vi "FPGA_fast cycles-4.vi"() -> ()   [LabVIEW 2010]
uses:
  fast cycles/FPGA_run-states.ctl
  <vilib>/rvi/DataTransferAndStorage/Container/XNode/niFpgaContainer.xnode
  <vilib>/eio/EIONode/EIONode.xnode
  <vilib>/rvi/eio/nirviEIOImplementation/nirviEIOImplementation.xnode
  <vilib>/rvi/eio/common/nirviEmuClasses.ctl
  <vilib>/rvi/FIFO/Fifo_Resource/nirvififoEmulationSetSize.vi
  <vilib>/rvi/DataTransferAndStorage/Container/Common/niFpgaContainerGetUniqueNameForEmu.vi
  <vilib>/rvi/Memory/Memory_Emulation/nirvimemoryEmulationManagerCache_GetValue.vi
  <vilib>/rvi/Memory/Memory_Emulation/nirvimemoryEmulationManagerCache_InsertValue.vi
  <vilib>/Utility/error.llb/Clear Errors.vi
  <vilib>/rvi/Memory/Memory_Emulation/nirvimemoryEmulationManagerCache_SetValue.vi
  <vilib>/rvi/eio/common/nirviEmuTemplateMethod_noerrors.vi
panel:
  out "ramp":bool
  out "trigDAC":bool
  in  "order in":u64=360850920143060992
  in  "get order":bool
  in  "Stop seq 2":bool=TRUE
  in  "stop on sample count":bool
  in  "samples":u16=1
  in  "pulse length":u16=100
  in  "Divider":u32=200000
  out "voltmeters trig":bool=TRUE
  in  "Stop seq":bool=TRUE
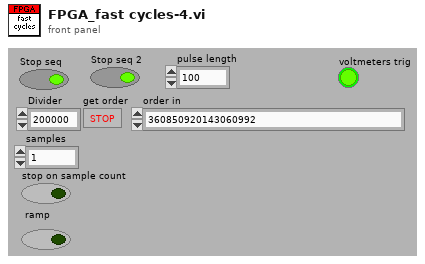
[diagram p1: front panel]
types:
  T1 = typedef "FPGA_run-states.ctl" = enum16{"stopped", "check", "reserve", "run", "release"}
  T2 = typedef "nirviEmuClasses.ctl" = enum16{"IO Read", "IO Write", "Method", "Property Read", "Property Write"}
  T3 = cluster{"Boolean array[0]":bool, "Boolean array[1]":bool, "Boolean array[2]":bool, "Boolean array[3]":bool, "Boolean array[4]":bool, "Boolean array[5]":bool, "Boolean array[6]":bool, "Boolean array[7]":bool, "Boolean array[8]":bool, "Boolean array[9]":bool, "Boolean array[10]":bool, "Boolean array[11]":bool, "Boolean array[12]":bool, "Boolean array[13]":bool, "Boolean array[14]":bool, "Boolean array[15]":bool}
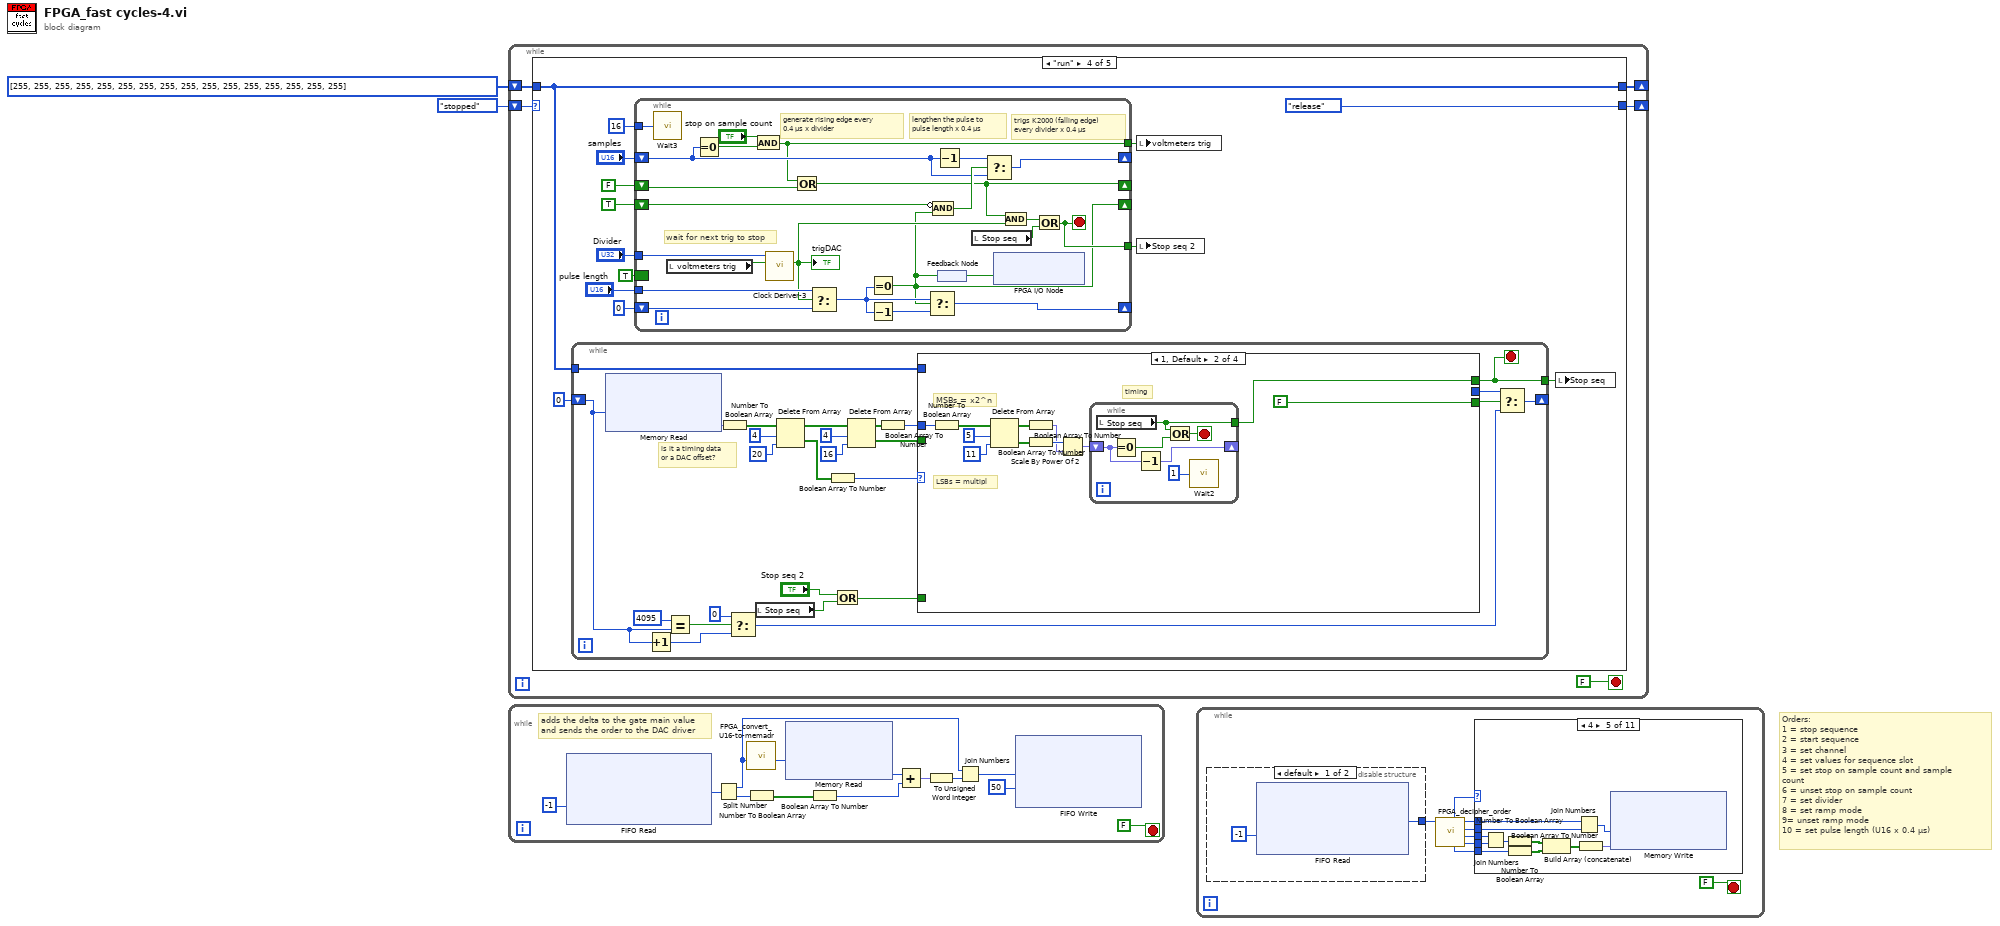
[diagram p0: block diagram]
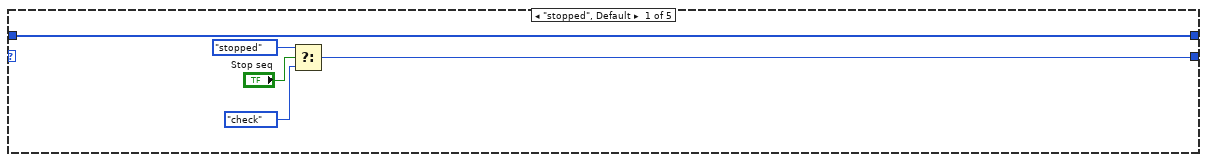
[diagram p2: hidden frame]
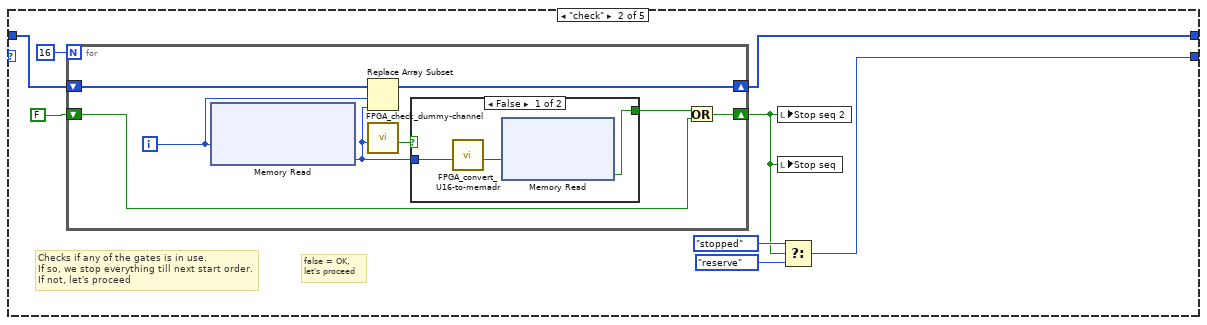
[diagram p3: hidden frame]
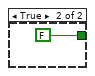
[diagram p4: hidden frame]
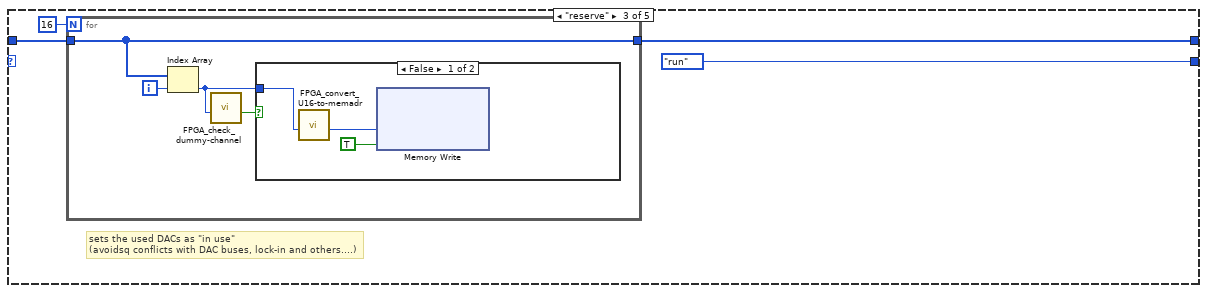
[diagram p5: hidden frame]
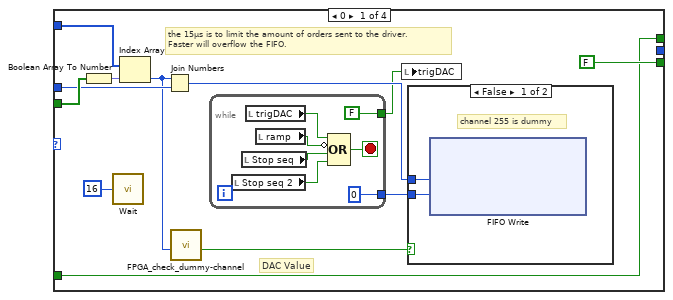
[diagram p7: hidden frame]
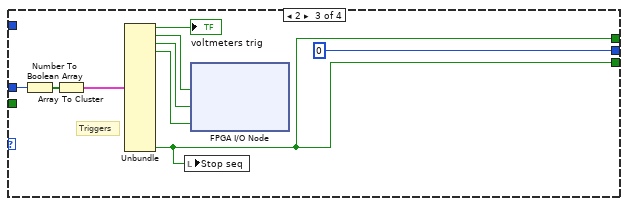
[diagram p9: hidden frame]
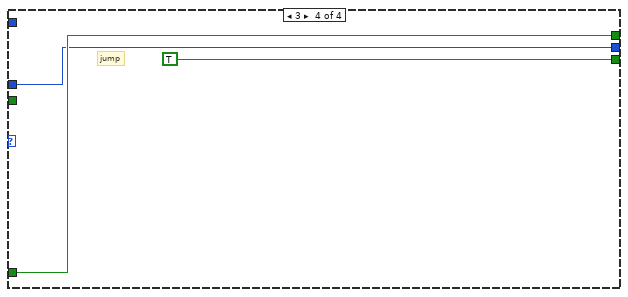
[diagram p10: hidden frame]
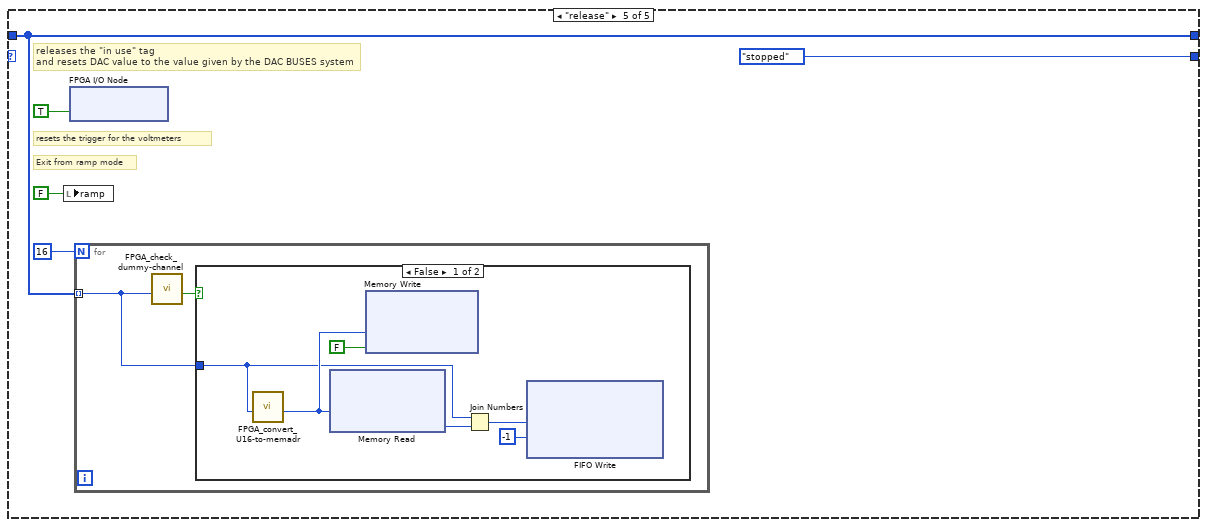
[diagram p11: hidden frame]
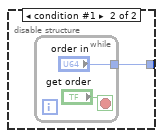
[diagram p13: hidden frame]
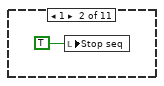
[diagram p15: hidden frame]
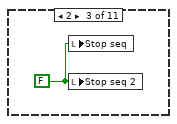
[diagram p16: hidden frame]
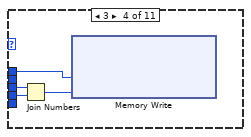
[diagram p17: hidden frame]
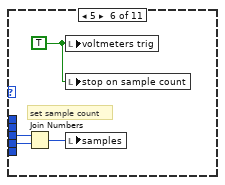
[diagram p18: hidden frame]
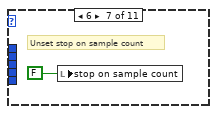
[diagram p19: hidden frame]
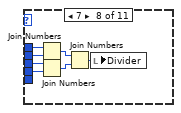
[diagram p20: hidden frame]
diagram:
  # "Orders:\n1 = stop sequence\n2 = start sequence\n3 = set channel\n4 = set values for sequence slot\n5 = set stop on sample count and sample count\n6 = unset stop on sample count\n7 = set divider\n8 = set ramp mode\n9= unset ramp mode\n10 = set pulse length (U16 x 0.4 µs)"
  n1 = while {
    shift-right: [w5] -> _
    shift-left: FPGA_run-states."stopped" ("run states") -> [w6]
    shift-right: [w3] -> _
    shift-left: u16[] [255, 255, 255, 255, 255, 255, 255, 255, 255, 255, 255, 255, 255, 255, 255, 255] -> [w4]
    stop <- FALSE stop-if-true
    n2 = case shown="\"run\"" w6 {
      tunnel: [w9 w13 FPGA_run-states."run" ("run states") FPGA_run-states."release" ("run states") FPGA_run-states."stopped" ("run states")] -> w5
      tunnel: [w8 w14 w285 w424 w757] -> w3
      tunnel: w4 -> [w8 w15 w286 w424 w757]
      frame "stopped", Default {
        n3 = Select(t=FPGA_run-states."stopped" ("run states"), s="Stop seq", f=FPGA_run-states."check" ("run states")) -> (s? t:f=w9:T1)
      }
      frame "check" {
        # "Checks if any of the gates is in use.\nIf so, we stop everything till next start order.\nIf not, let's proceed"
        # "false = OK,\nlet's proceed"
        n4 = for {
          N: 16 -> [_]
          shift-right: [w26] -> w16
          shift-left: FALSE ("Data") -> [w25]
          shift-right: [w24] -> w14
          shift-left: w15 -> [w23]
          i -> [w28]
          n5 = xnode ("Memory Read")("Address"=w28) -> ("Data"=w21:u16)  [unwired: 1 in, 1 out]
          n6 = Replace Array Subset(array=w23, new element=w21, index=w28) -> (w24:u16[])
          n7 = call "FPGA_check_dummy-channel.vi"("pan-channel"=w21) -> ("dummy?"=w22:bool)  [unwired: 10 out]
          n8 = case shown="False" w22 {
            tunnel: w21 -> [w157 _]
            tunnel: [w155 FALSE ("Data")] -> w27
            frame False {
              n9 = call "FPGA_convert_U16-to-memadr.vi"("Numeric"=w157) -> ("mem adr"=w156:u8)  [unwired: 10 out]
              n10 = xnode ("Memory Read")("Address"=w156) -> ("Data"=w155:bool)  [unwired: 1 in, 1 out]
            }
            frame True {
            }
          }
          n11 = Or(x=w27, y=w25) -> (x .or. y?=w26:bool)
        }
        n12 = local write "Stop seq 2"(w16) -> ()
        n13 = local write "Stop seq"(w16) -> ()
        n14 = Select(t=FPGA_run-states."stopped" ("run states"), s=w16, f=FPGA_run-states."reserve" ("run states")) -> (s? t:f=w13:T1)
      }
      frame "reserve" {
        # "sets the used DACs as \"in use\"\n(avoidsq conflicts with DAC buses, lock-in and others....)"
        n15 = for {
          N: 16 -> [_]
          tunnel: w286 -> [w291]
          tunnel: [w291] -> w285
          i -> [w292]
          n16 = Index Array(array=w291, index=w292) -> (element=w290:u16)
          n17 = call "FPGA_check_dummy-channel.vi"("pan-channel"=w290) -> ("dummy?"=w289:bool)  [unwired: 10 out]
          n18 = case shown="False" w289 {
            tunnel: w290 -> [w293 _]
            frame False {
              n19 = call "FPGA_convert_U16-to-memadr.vi"("Numeric"=w293) -> ("mem adr"=w295:u8)  [unwired: 10 out]
              n20 = xnode ("Memory Write")("Address"=w295, "Data"=TRUE) -> ()  [unwired: 1 in, 1 out]
            }
            frame True {
            }
          }
        }
      }
      frame "run" {
        n21 = while {
          shift-right: [w478] -> _
          shift-left: u16 0 ("t") -> [w490]
          tunnel: [w471] -> w426
          tunnel: w424 -> [w470]
          stop <- w471 stop-if-true
          # "is it a timing data\nor a DAC offset?"
          n22 = xnode ("Memory Read")("Address"=w490) -> ("Data"=w489:fxp<+,24,24>)  [unwired: 1 in, 1 out]
          n23 = Increment(x=w490) -> (x+1=w492:u16)
          n24 = Equal?(x=u16 4095, y=w490) -> (x = y?=w494:bool)
          n25 = Number To Boolean Array(number=w489) -> (Boolean array=w488:bool[])
          n26 = Select(t=u16 0, s=w494, f=w492) -> (s? t:f=w491:u16)
          n27 = local read "Stop seq"() -> (w475:bool)
          n28 = Delete From Array(array=w488, length=4, index=20) -> (deleted portion=w481:bool[], array with subset deleted=w485:bool[])
          n29 = Boolean Array To Number(Boolean array=w481) -> (number=w479:u8)
          n30 = Or(x="Stop seq 2", y=w475) -> (x .or. y?=w473:bool)
          n31 = Delete From Array(array=w485, length=4, index=16) -> (deleted portion=w482:bool[], array with subset deleted=w483:bool[])
          n32 = Boolean Array To Number(Boolean array=w483) -> (number=w474:u16)
          n33 = case shown="1, Default" w479 {
            tunnel: w474 -> [w631 w704 w719 w753]
            tunnel: w482 -> [w633 _ _ _]
            tunnel: [FALSE ("Stop seq") FALSE ("Stop seq") w713 TRUE ("Stop seq")] -> w477
            tunnel: [_ _ u16 0 w753] -> w476
            tunnel: [w627 w694 w713 w754] -> w471
            tunnel: w473 -> [w627 _ _ w754]
            tunnel: w470 -> [w625 _ _ _]
            frame 0 {
              # "the 15µs is to limit the amount of orders sent to the driver.\nFaster will overflow the FIFO."
              # "DAC Value"
              n34 = Boolean Array To Number(Boolean array=w633) -> (number=w632:fxp<+,4,4>)
              n35 = call "Wait"("Count(uSec)"=u8 16) -> ()  [unwired: 1 out]
              n36 = Index Array(array=w625, index=w632) -> (element=w623:u16)
              n37 = Join Numbers(hi=w623, lo=w631) -> ((hi.lo)=w630:u32)
              n38 = call "FPGA_check_dummy-channel.vi"("pan-channel"=w623) -> ("dummy?"=w624:bool)  [unwired: 10 out]
              n39 = while {
                tunnel: [0 ("Timeout")] -> w626
                tunnel: [FALSE ("Stop seq 3")] -> w622
                stop <- w688 stop-if-true
                n40 = local read "Stop seq 2"() -> (w691:bool)
                n41 = local read "Stop seq"() -> (w692:bool)
                n42 = local read "trigDAC"() -> (w689:bool)
                n43 = local read "ramp"() -> (w690:bool)
                n44 = Compound Arithmetic op=OR(w689, invert w690, w692, w691) -> (w688:bool)
              }
              n45 = local write "trigDAC"(w622) -> ()
              n46 = case shown="False" w624 {
                tunnel: w630 -> [w635 _]
                tunnel: w626 -> [w634 _]
                frame False {
                  # "channel 255 is dummy"
                  n47 = xnode ("FIFO Write")("Element"=w635, "Timeout"=w634) -> ()  [unwired: 1 in, 2 out]
                }
                frame True {
                }
              }
            }
            frame 1, Default {
              # "MSBs = x2^n"
              # "LSBs = multipl"
              # "timing"
              n48 = Number To Boolean Array(number=w704) -> (Boolean array=w703:bool[])
              n49 = Delete From Array(array=w703, length=5 ("longueur"), index=11 ("indice")) -> (deleted portion=w699:bool[], array with subset deleted=w700:bool[])
              n50 = Boolean Array To Number ("Tableau de booléens en nombre")(Boolean array=w700) -> (number=w697:fxp<+,37,37>)
              n51 = Boolean Array To Number ("Tableau de booléens en nombre")(Boolean array=w699) -> (number=w698:u8)
              n52 = Scale By Power Of 2(n=w698, x=w697) -> (x*2^n=w696:fxp<+,37,37>)
              n53 = while {
                shift-right: [w710] -> _
                shift-left: w696 -> [w709]
                tunnel: [w705] -> w694
                stop <- w708 stop-if-true
                n54 = local read "Stop seq"() -> (w705:bool)
                n55 = Equal To 0?(x=w709) -> (x = 0?=w706:bool)
                n56 = Decrement ("Décrémenter")(x=w709) -> (x-1=w710:fxp<+,37,37>)
                n57 = Or(x=w705, y=w706) -> (x .or. y?=w708:bool)
                n58 = call "Wait2"("Count(uSec)"=u8 1) -> ()  [unwired: 1 out]
              }
            }
            frame 2 {
              # "Triggers"
              n59 = Number To Boolean Array(number=w719) -> (Boolean array=w718:bool[])
              n60 = Array To Cluster(array=w718) -> (cluster=w717:T3)
              n61 = Unbundle(w717) -> ("Boolean array[0]"=→"voltmeters trig":bool, "Boolean array[1]"=w716:bool, "Boolean array[2]"=w715:bool, "Boolean array[3]"=w712:bool, "Boolean array[15]"=w713:bool)  [unwired: 11 out]
              n62 = local write "Stop seq"(w713) -> ()
              n63 = xnode "FPGA I/O Node"("Port9/DIO2"=w716, "Port9/DIO3"=w715, "Port9/DIO4"=w712) -> ()  [unwired: 3 in, 3 out]
            }
            frame 3 {
              # "jump"
            }
          }
          n64 = Select(t=w476, s=w477, f=w491) -> (s? t:f=w478:u16)
        }
        n65 = while {
          tunnel: "Divider" -> [w458]
          tunnel: "pulse length" -> [w456]
          shift-right: [w453] -> _
          shift-left: u16 0 ("pulse length") -> [w455]
          shift-right: [w450] -> _
          shift-left: "samples" -> [w449]
          shift-right: [w435] -> _
          shift-left: TRUE -> [w436]
          tunnel: u8 16 ("Count(Ticks)") -> [w448]
          tunnel: [w444] -> w428
          tunnel: [w445] -> w427
          shift-right: [w440] -> _
          shift-left: FALSE -> [w442]
          border: TRUE -> [_]
          stop <- w445 stop-if-true
          # "wait for next trig to stop"
          # "trigs K2000 (falling edge)\nevery divider x 0.4 µs"
          # "lengthen the pulse to\npulse length x 0.4 µs"
          # "generate rising edge every\n0.4 µs x divider"
          n66 = call "Wait3"("Count(Ticks)"=w448) -> ()  [unwired: 1 out]
          n67 = local read "voltmeters trig"() -> (w446:bool)
          n68 = Equal To 0?(x=w449) -> (x = 0?=w438:bool)
          n69 = And(x="stop on sample count", y=w438) -> (x .and. y?=w444:bool)
          n70 = call "Clock Deriver-3.vi"("reset"=w446, "Divisor"=w458) -> ("Clock Out"=w439:bool)  [unwired: 1 in, 8 out]
          "trigDAC" <- w439
          n71 = Or(x=w444, y=w442) -> (x .or. y?=w440:bool)
          n72 = Select(t=w456, s=w439, f=w455) -> (s? t:f=w454:u16)
          n73 = Equal To 0?(x=w454) -> (x = 0?=w435:bool)
          n74 = Decrement(x=w454) -> (x-1=w457:u16)
          n75 = Select(t=w454, s=w435, f=w457) -> (s? t:f=w453:u16)
          n76 = Compound Arithmetic op=AND(invert w436, w435) -> (w452:bool)
          n77 = Decrement(x=w449) -> (x-1=w451:u16)
          n78 = feedback-in #1(w435) -> ()
          n79 = feedback #1() -> (w441:bool)
          n80 = local read "Stop seq"() -> (w447:bool)
          n81 = Select(t=w451, s=w452, f=w449) -> (s? t:f=w450:u16)
          n82 = xnode "FPGA I/O Node"("Port9/DIO1"=w441) -> ()  [unwired: 1 in, 1 out]
          n83 = And(x=w440, y=w439) -> (x .and. y?=w443:bool)
          n84 = Or(x=w443, y=w447) -> (x .or. y?=w445:bool)
        }
        n85 = local write "voltmeters trig"(w428) -> ()
        n86 = local write "Stop seq 2"(w427) -> ()
        n87 = local write "Stop seq"(w426) -> ()
      }
      frame "release" {
        # "Exit from ramp mode"
        # "resets the trigger for the voltmeters"
        # "releases the \"in use\" tag\nand resets DAC value to the value given by the DAC BUSES system"
        n88 = local write "ramp"(FALSE ("ramp")) -> ()
        n89 = xnode "FPGA I/O Node"("Port9/DIO1"=TRUE) -> ()  [unwired: 1 in, 1 out]
        n90 = for {
          N: 16 -> [_]
          tunnel: w757 -> [w772] mode=indexing
          n91 = call "FPGA_check_dummy-channel.vi"("pan-channel"=w772) -> ("dummy?"=w773:bool)  [unwired: 10 out]
          n92 = case shown="False" w773 {
            tunnel: w772 -> [w774 _]
            frame False {
              n93 = call "FPGA_convert_U16-to-memadr.vi"("Numeric"=w774) -> ("mem adr"=w778:u8)  [unwired: 10 out]
              n94 = xnode ("Memory Read")("Address"=w778) -> ("Data"=w776:u16)  [unwired: 1 in, 1 out]
              n95 = xnode ("Memory Write")("Address"=w778, "Data"=FALSE) -> ()  [unwired: 1 in, 1 out]
              n96 = Join Numbers(hi=w774, lo=w776) -> ((hi.lo)=w777:u32)
              n97 = xnode ("FIFO Write")("Element"=w777, "Timeout"=-1) -> ()  [unwired: 1 in, 2 out]
            }
            frame True {
            }
          }
        }
      }
    }
  }
  n98 = while {
    stop <- FALSE stop-if-true
    # "adds the delta to the gate main value\nand sends the order to the DAC driver"
    n99 = xnode ("FIFO Read")("Timeout"=-1) -> ("Element"=w1093:u32)  [unwired: 1 in, 2 out]
    n100 = Split Number(x=w1093) -> (hi(x)=w1083:u16, lo(x)=w1085:u16)
    n101 = call "FPGA_convert_U16-to-memadr.vi"("Numeric"=w1083) -> ("mem adr"=w1084:u8)  [unwired: 10 out]
    n102 = Number To Boolean Array(number=w1085) -> (Boolean array=w1090:bool[])
    n103 = xnode ("Memory Read")("Address"=w1084) -> ("Data"=w1092:u16)  [unwired: 1 in, 1 out]
    n104 = Boolean Array To Number(Boolean array=w1090) -> (number=w1089:i16)
    n105 = Add(x=w1092, y=w1089) -> (x+y=w1088:fxp<+,16,16>)
    n106 = To Unsigned Word Integer(number=w1088) -> (unsigned 16bit integer=w1086:u16)
    n107 = Join Numbers(hi=w1083, lo=w1086) -> ((hi.lo)=w1087:u32)
    n108 = xnode ("FIFO Write")("Element"=w1087, "Timeout"=50) -> ()  [unwired: 1 in, 2 out]
  }
  n109 = while {
    stop <- FALSE stop-if-true
    n110 = disable-structure shown="default" {
      disable-tunnel: [w1331 w1384] -> w1329
      frame condition #0 (active) {
        n111 = xnode ("FIFO Read")("Timeout"=-1) -> ("Element"=w1331:u64)  [unwired: 1 in, 2 out]
      }
      frame condition #1 {
        n112 = while {
          tunnel: ["order in"] -> w1384
          stop <- "get order" stop-if-true
        }
      }
    }
    n113 = call "FPGA_decipher_order.vi"("order in"=w1329) -> ("data 1"=w1327:u8, "data 2"=w1326:u8, "data 3"=w1324:u8, "data 4"=w1325:u8, "RFU 2"=w1323:u8, "order out"=w1328:u8)  [unwired: 5 out]
    n114 = case shown="4" w1328 {
      tunnel: w1327 -> [_ _ _ w1390 w1528 w1656 _ w1662 w1668 _ w1674]
      tunnel: w1326 -> [_ _ _ w1391 w1527 w1657 _ w1663 w1667 _ w1673]
      tunnel: w1325 -> [_ _ _ w1392 w1521 _ _ w1665 _ _ _]
      tunnel: w1324 -> [_ _ _ _ w1520 _ _ w1664 _ _ _]
      tunnel: w1323 -> [_ _ _ _ w1518 _ _ _ _ _ _]
      frame 0, Default {
      }
      frame 1 {
        n115 = local write "Stop seq"(TRUE ("Stop seq")) -> ()
      }
      frame 2 {
        w1388 = FALSE ("Stop seq")
        n116 = local write "Stop seq"(w1388) -> ()
        n117 = local write "Stop seq 2"(w1388) -> ()
      }
      frame 3 {
        n118 = Join Numbers(hi=w1391, lo=w1390) -> ((hi.lo)=w1389:u16)
        n119 = xnode ("Memory Write")("Address"=w1392, "Data"=w1389) -> ()  [unwired: 1 in, 1 out]
      }
      frame 4 {
        n120 = Join Numbers(hi=w1527, lo=w1528) -> ((hi.lo)=w1526:u16)
        n121 = Number To Boolean Array(number=w1526) -> (Boolean array=w1525:bool[])
        n122 = Number To Boolean Array(number=w1518) -> (Boolean array=w1524:bool[])
        n123 = Build Array (concatenate)(w1525, w1524) -> (w1523:bool[])
        n124 = Join Numbers(hi=w1521, lo=w1520) -> ((hi.lo)=w1522:u16)
        n125 = Boolean Array To Number(Boolean array=w1523) -> (number=w1519:fxp<+,24,24>)
        n126 = xnode ("Memory Write")("Address"=w1522, "Data"=w1519) -> ()  [unwired: 1 in, 1 out]
      }
      frame 5 {
        w1654 = TRUE
        # "set sample count"
        n127 = Join Numbers(hi=w1657, lo=w1656) -> ((hi.lo)=w1655:u16)
        n128 = local write "voltmeters trig"(w1654) -> ()
        n129 = local write "stop on sample count"(w1654) -> ()
        n130 = local write "samples"(w1655) -> ()
      }
      frame 6 {
        # "Unset stop on sample count"
        n131 = local write "stop on sample count"(FALSE) -> ()
      }
      frame 7 {
        n132 = Join Numbers(hi=w1665, lo=w1664) -> ((hi.lo)=w1661:u16)
        n133 = Join Numbers(hi=w1663, lo=w1662) -> ((hi.lo)=w1660:u16)
        n134 = Join Numbers(hi=w1661, lo=w1660) -> ((hi.lo)=w1659:u32)
        n135 = local write "Divider"(w1659) -> ()
      }
      frame 8 {
        w1670 = TRUE
        n136 = Join Numbers(hi=w1667, lo=w1668) -> ((hi.lo)=w1669:u16)
        n137 = local write "trigDAC"(FALSE ("trigDAC")) -> ()
        n138 = local write "stop on sample count"(w1670) -> ()
        n139 = local write "voltmeters trig"(w1670) -> ()
        n140 = local write "samples"(w1669) -> ()
        "ramp" <- w1670
      }
      frame 9 {
        w1671 = FALSE
        n141 = local write "ramp"(w1671) -> ()
        n142 = local write "stop on sample count"(w1671) -> ()
      }
      frame 10 {
        # "set the length of"
        n143 = Join Numbers(hi=w1673, lo=w1674) -> ((hi.lo)=w1672:u16)
        n144 = local write "pulse length"(w1672) -> ()
      }
    }
  }
